vi "0x53_Write_table_data.vi"(8 "error in":errorcluster, 9 "Номер табличного параметра 2":i32, 10 "ArrayIn":sgl[][](array[numeric]), 11 "paramUnicorn":T1={"conParam"={"ReadIntParam"=TRUE, "ReadDescrParam"=FALSE, "ReadFloatParam"=TRUE, "debug"=FALSE, "ReadJSON"=TRUE, "IP_address"="192.168.1.216", "N_attempts"=3, "type_con"=enum."TCP", "MB_address"=1, "VISA"="COM1", "connection ID"=refnum, "nameDevices"="", "timeout"=3000, "port"=2000, "type_version"="0F0C0001", "baud_rate"=115200, "VersionControl"=TRUE, "TCP_conn"=TRUE, "WindowSize"=700}, "Param"={"NumParam"={"NTelem"=201, "NInt"=16, "NFloat"=10, "NTable"=2}, "ParamInt"=[{"ID"="Режим работы", "Num"=0, "Name"="", "Type"="", "Enum"="", "Desc"="", "Unit"="", "Access"="", "FormatStr"="", "Min"=0, "Max"=0}, {"ID"="", "Num"=0, "Name"="", "Type"="", "Enum"="", "Desc"="", "Unit"="", "Access"="", "FormatStr"="", "Min"=0, "Max"=0}, {"ID"="", "Num"=0, "Name"="", "Type"="", "Enum"="", "Desc"="", "Unit"="", "Access"="", "FormatStr"="", "Min"=0, "Max"=0}, {"ID"="", "Num"=0, "Name"="", "Type"="", "Enum"="", "Desc"="", "Unit"="", "Access"="", "FormatStr"="", "Min"=0, "Max"=0}, {"ID"="", "Num"=0, "Name"="", "Type"="", "Enum"="", "Desc"="", "Unit"="", "Access"="", "FormatStr"="", "Min"=0, "Max"=0}, {"ID"="", "Num"=0, "Name"="", "Type"="", "Enum"="", "Desc"="", "Unit"="", "Access"="", "FormatStr"="", "Min"=0, "Max"=0}, {"ID"="ModeWork", "Num"=0, "Name"="", "Type"="", "Enum"="", "Desc"="", "Unit"="", "Access"="", "FormatStr"="", "Min"=0, "Max"=0}], "Telemetry"=[], "Table"=[], "ParamFloat"=[]}}) -> (0 "error out":errorcluster, 2 "Ответ":string, 3 "paramUnicorn 2":T1={"conParam"={"ReadIntParam"=TRUE, "ReadDescrParam"=FALSE, "ReadFloatParam"=TRUE, "debug"=FALSE, "ReadJSON"=TRUE, "IP_address"="192.168.1.216", "N_attempts"=3, "type_con"=enum."TCP", "MB_address"=1, "VISA"="COM1", "connection ID"=refnum, "nameDevices"="", "timeout"=3000, "port"=2000, "type_version"="0F0C0001", "baud_rate"=115200, "VersionControl"=TRUE, "TCP_conn"=TRUE, "WindowSize"=700}, "Param"={"NumParam"={"NTelem"=201, "NInt"=16, "NFloat"=10, "NTable"=2}, "ParamInt"=[{"ID"="Режим работы", "Num"=0, "Name"="", "Type"="", "Enum"="", "Desc"="", "Unit"="", "Access"="", "FormatStr"="", "Min"=0, "Max"=0}, {"ID"="", "Num"=0, "Name"="", "Type"="", "Enum"="", "Desc"="", "Unit"="", "Access"="", "FormatStr"="", "Min"=0, "Max"=0}, {"ID"="", "Num"=0, "Name"="", "Type"="", "Enum"="", "Desc"="", "Unit"="", "Access"="", "FormatStr"="", "Min"=0, "Max"=0}, {"ID"="", "Num"=0, "Name"="", "Type"="", "Enum"="", "Desc"="", "Unit"="", "Access"="", "FormatStr"="", "Min"=0, "Max"=0}, {"ID"="", "Num"=0, "Name"="", "Type"="", "Enum"="", "Desc"="", "Unit"="", "Access"="", "FormatStr"="", "Min"=0, "Max"=0}, {"ID"="", "Num"=0, "Name"="", "Type"="", "Enum"="", "Desc"="", "Unit"="", "Access"="", "FormatStr"="", "Min"=0, "Max"=0}, {"ID"="ModeWork", "Num"=0, "Name"="", "Type"="", "Enum"="", "Desc"="", "Unit"="", "Access"="", "FormatStr"="", "Min"=0, "Max"=0}], "Telemetry"=[], "Table"=[], "ParamFloat"=[]}}, 5 "Сообщение об ошибке":bool)   [LabVIEW 2017, in "LV_Unicorn.lvlib"]
uses:
  LV_Unicorn.lvlib
  Control/unicorn_Param.ctl
  Control/unicorn_conn.ctl
  Control/unicorn_JSON.ctl
  Control/unicorn_ParamInt.ctl
  Control/unicorn_Telemetry.ctl
  Control/unicorn_Table.ctl
  Control/unicorn_ParamFloat.ctl
panel:
  out "Slide":u8(slide) caption="Запись табличного параметра" scale=0.0..100.0
  out "Size":i32
  out "Array":string[](array[string])
  out "length 2":i32
  out "lengthData":i32
  out "String out":string
  out "кол-во считанных байт тела запрошенного параметра":i32
  out "Начальное смещение в байтах":i32
  out "Номер табличного параметра":i32
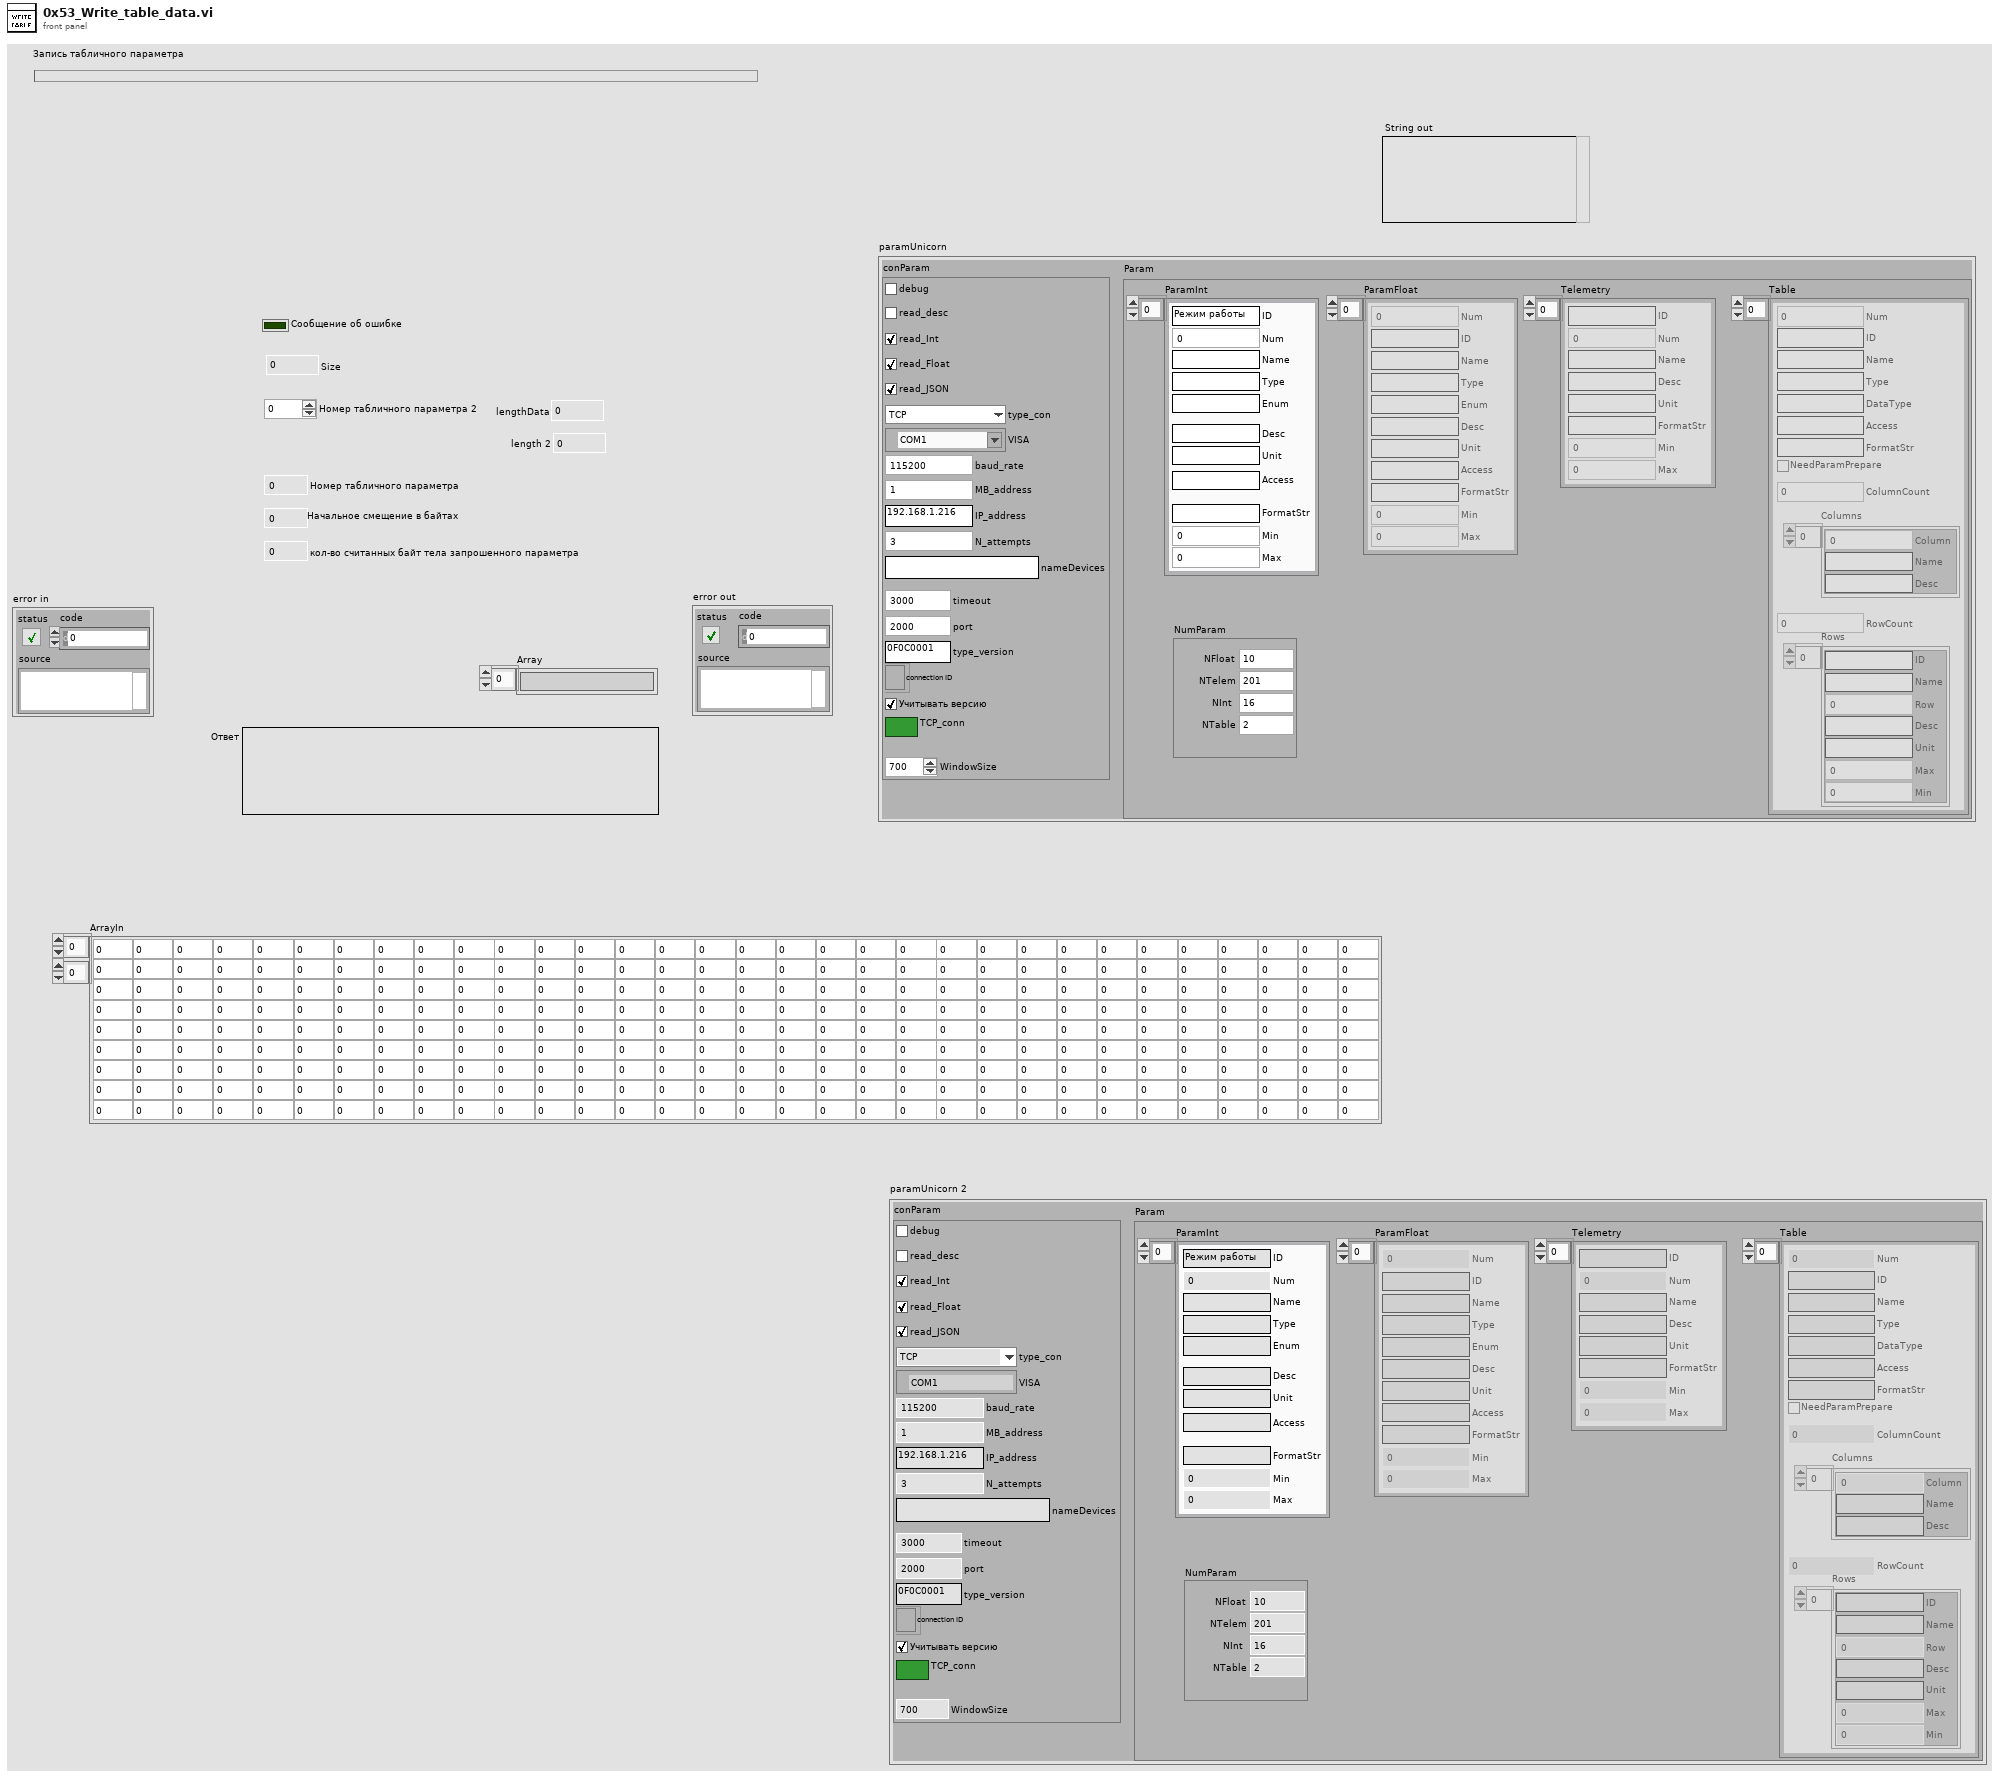
[diagram p1: front panel]
types:
  T1 = typedef "LV_Unicorn.lvlib/unicorn_Param.ctl" = cluster{"conParam":T2, "Param":T3}
  T2 = typedef "LV_Unicorn.lvlib/unicorn_conn.ctl" = cluster{"ReadIntParam":bool, "ReadDescrParam":bool, "ReadFloatParam":bool, "debug":bool, "ReadJSON":bool, "IP_address":string, "N_attempts":i32, "type_con":enum16{"Serial", "TCP"}, "MB_address":i32, "VISA":refnum<visa-resource-name>, "connection ID":refnum<k5>, "nameDevices":string, "timeout":i32, "port":u16, "type_version":string, "baud_rate":u32, "VersionControl":bool, "TCP_conn":bool, "WindowSize":i32}
  T3 = typedef "LV_Unicorn.lvlib/unicorn_JSON.ctl" = cluster{"NumParam":cluster{"NTelem":i32, "NInt":i32, "NFloat":i32, "NTable":i32}, "ParamInt":T4, "Telemetry":T5, "Table":T6, "ParamFloat":T7}
  T4 = typedef "LV_Unicorn.lvlib/unicorn_ParamInt.ctl" = cluster{"ID":string, "Num":i32, "Name":string, "Type":string, "Enum":string, "Desc":string, "Unit":string, "Access":string, "FormatStr":string, "Min":i32, "Max":i32}[]
  T5 = typedef "LV_Unicorn.lvlib/unicorn_Telemetry.ctl" = cluster{"ID":string, "Num":i32, "Name":string, "Desc":string, "Unit":string, "FormatStr":string, "Min":i32, "Max":i32}[]
  T6 = typedef "LV_Unicorn.lvlib/unicorn_Table.ctl" = cluster{"Num":i32, "Access":string, "ColumnCount":i32, "NeedParamPrepare":bool, "Columns":cluster{"Column":i32, "Desc":string, "Name":string}[], "DataType":string, "FormatStr":string, "ID":string, "Name":string, "RowCount":i32, "Rows":cluster{"Desc":string, "ID":string, "Max":i32, "Min":i32, "Name":string, "Row":i32, "Unit":string}[], "Type":string}[]
  T7 = typedef "LV_Unicorn.lvlib/unicorn_ParamFloat.ctl" = cluster{"ID":string, "Num":i32, "Name":string, "Type":string, "Enum":string, "Desc":string, "Unit":string, "Access":string, "FormatStr":string, "Min":sgl, "Max":sgl}[]
  T8 = cluster{"Начальное смещение в байтах":i32, "Номер табличного параметра":i32, "Шаг":i32, "Размер слова":i32}
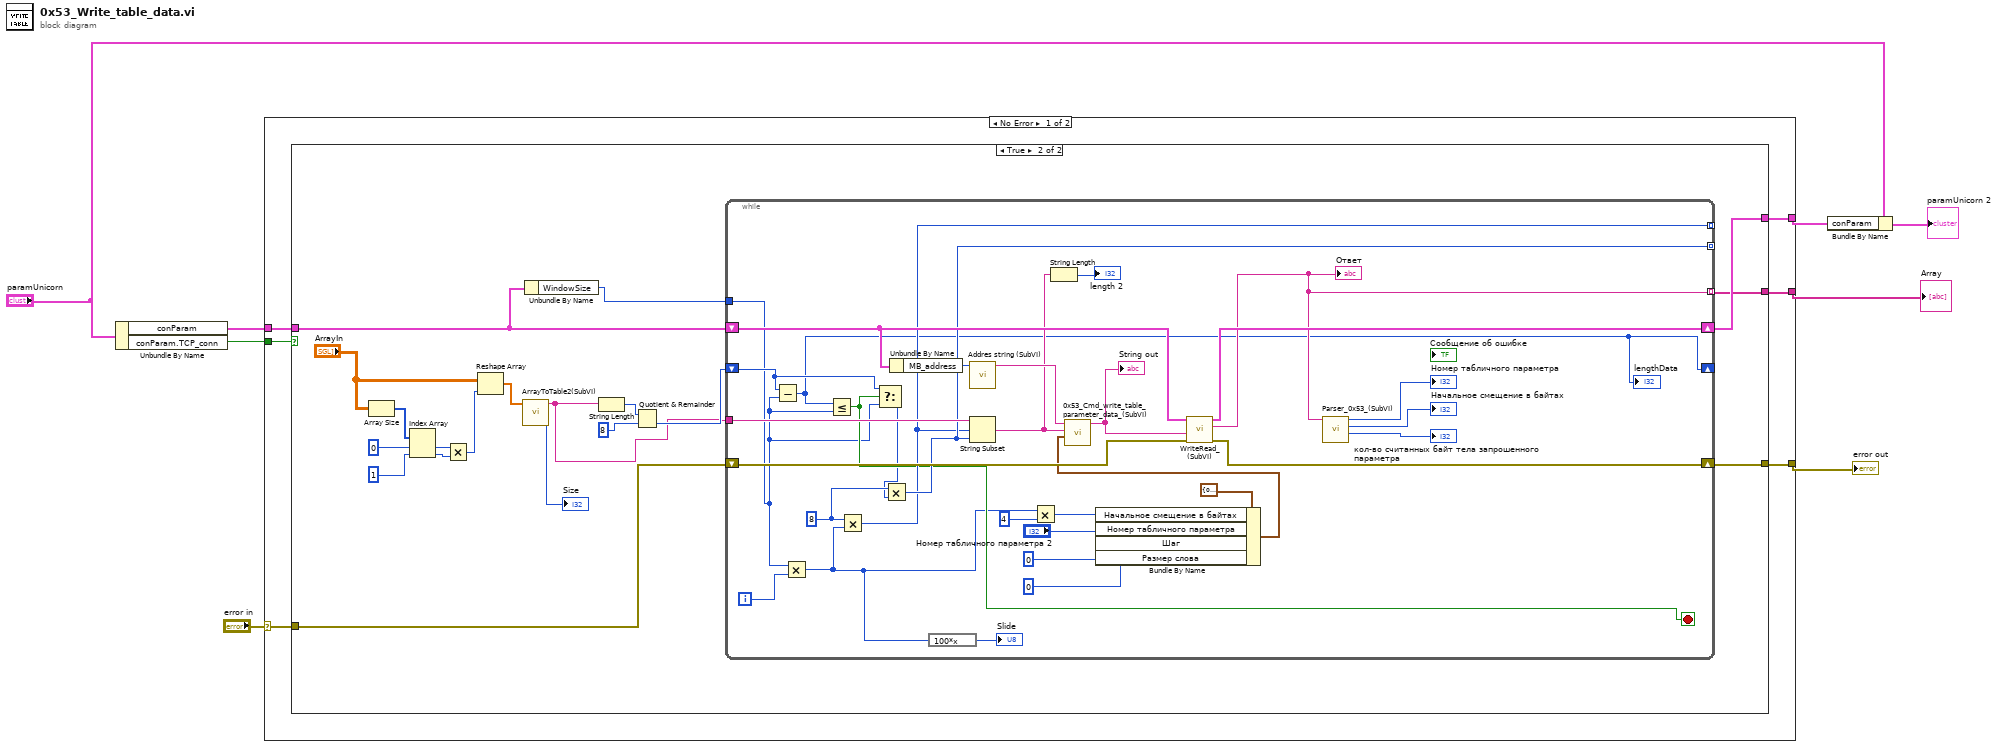
[diagram p0: block diagram]
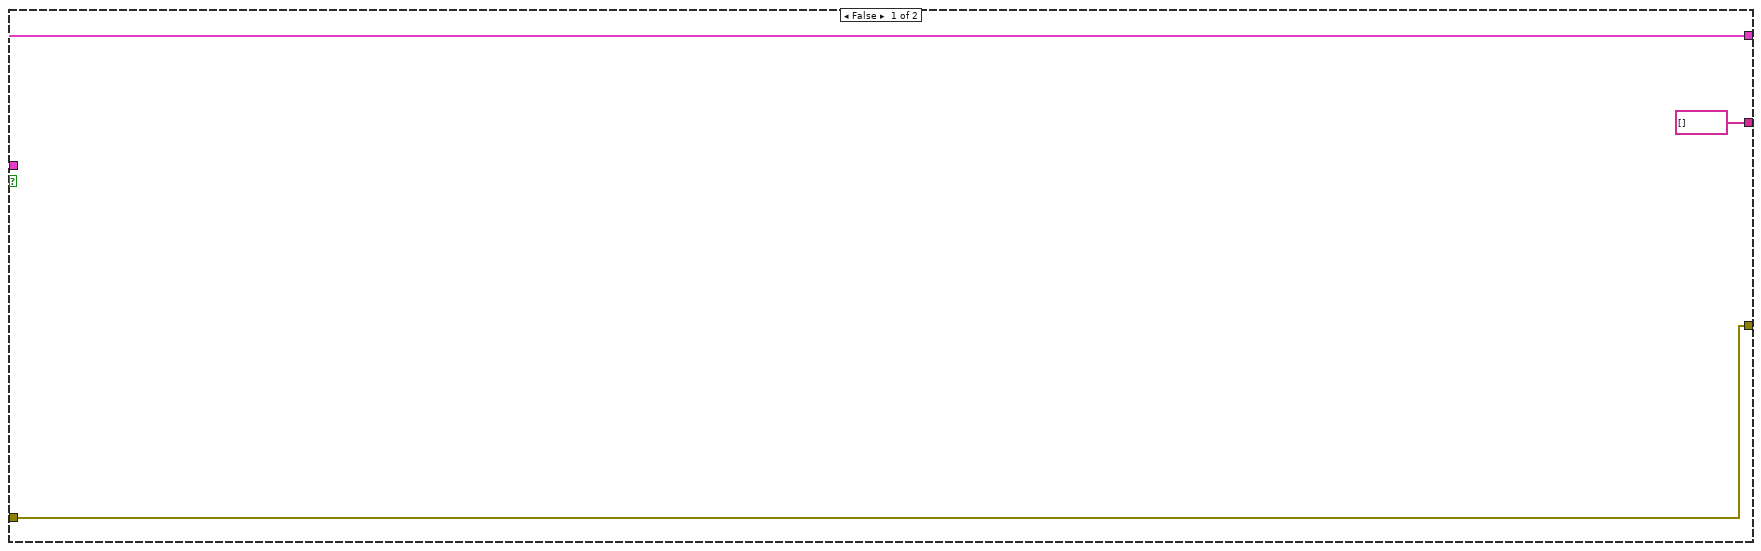
[diagram p2: hidden frame]
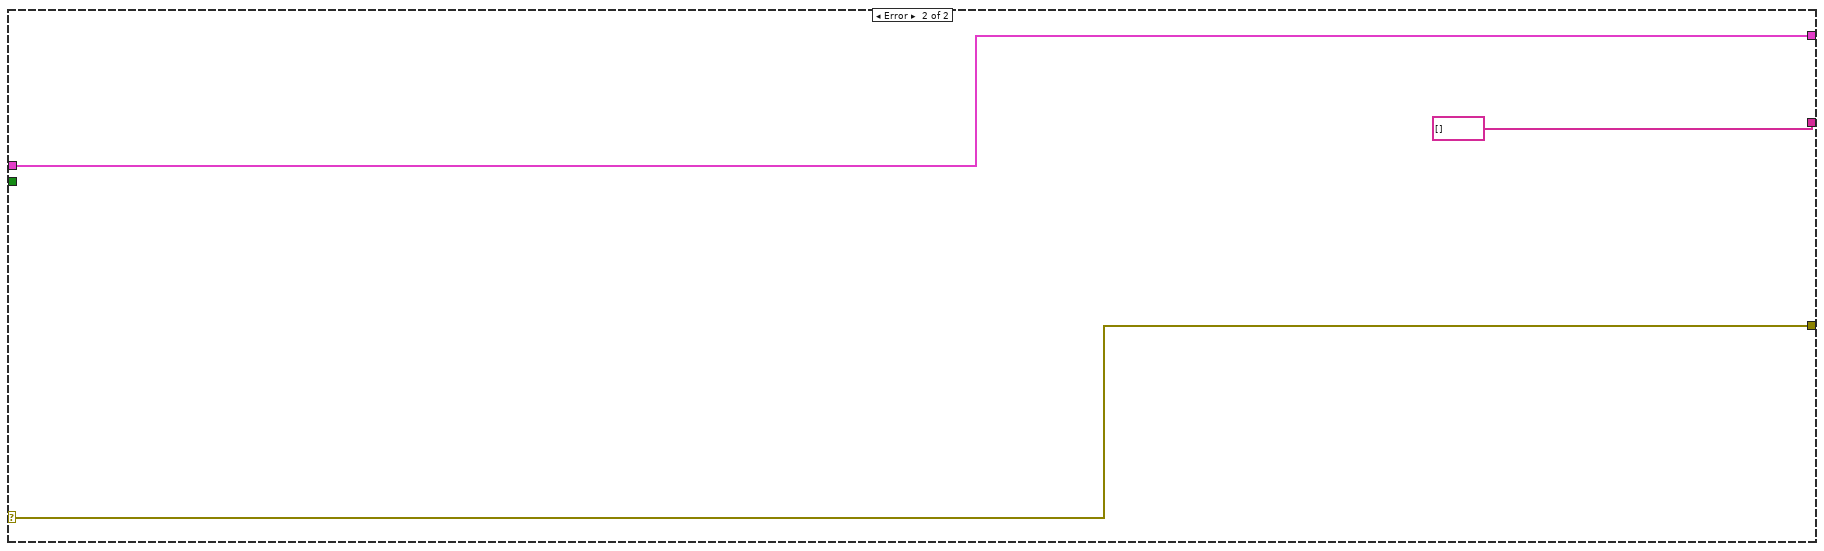
[diagram p3: hidden frame]
diagram:
  n1 = Unbundle By Name("paramUnicorn") -> ("conParam"=w6:T2, "conParam.TCP_conn"=w1:bool)
  n2 = case shown="No Error" "error in" {
    selector: "error in" -> [w12 w70]
    tunnel: w6 -> [w11 w71]
    tunnel: [w14 w71] -> w4
    tunnel: [w13 w70] -> w8
    tunnel: [w10 string[] []] -> w2
    tunnel: w1 -> [w9 _]
    frame No Error {
      n3 = case shown="True" w9 {
        tunnel: [w16 w36] -> w14
        tunnel: [w17 w35] -> w13
        tunnel: w12 -> [w17 w34]
        tunnel: w11 -> [w16 w19]
        tunnel: [string[] [] w20] -> w10
        frame False {
        }
        frame True {
          n4 = Array Size(array="ArrayIn") -> (size(s)=w30:i32[])
          n5 = Index Array(array=w30, index #1=0 ("index"), index #2=1 ("index")) -> (element #1=w31:i32, element #2=w32:i32)
          n6 = Multiply(x=w31, y=w32) -> (x*y=w33:i32)
          n7 = Reshape Array("ArrayIn", w33) -> (w28:sgl[])
          n8 = call "ArrayToTable2(SubVI).vi"("Table1D"=w28) -> ("Size"=→"Size":i32, "String"=w21:string)  [unwired: 9 in]
          n9 = Unbundle By Name(w19) -> ("WindowSize"=w18:i32)
          n10 = String Length(string=w21) -> (length=w27:i32)
          n11 = Quotient & Remainder(x=w27, y=8) -> (floor(x/y)=w22:i32)  [unwired: 1 out]
          n12 = while {
            shift-right: [w67] -> w35
            shift-left: w34 -> [w66]
            shift-right: [w68] -> w36
            shift-left: w19 -> [w65]
            tunnel: w21 -> [w59]
            tunnel: [w57] -> w20 mode=indexing
            shift-right: [w39] -> _
            shift-left: w22 -> [w43]
            tunnel: [w45] -> _ mode=indexing
            tunnel: [w50] -> _ mode=indexing
            tunnel: w18 -> [w37]
            i -> [w47]
            stop <- w44 stop-if-true
            w46 = 8 ("y")
            n13 = Subtract(x=w43, y=w37) -> (x-y=w39:i32)
            "lengthData" <- w39
            n14 = Multiply(x=w37, y=w47) -> (x*y=w38:i32)
            n15 = Less Or Equal?(x=w39, y=w37) -> (x <= y?=w44:bool)
            n16 = Multiply(x=w46, y=w38) -> (x*y=w45:i32)
            n17 = Select(t=w43, s=w44, f=w37) -> (s? t:f=w42:i32)
            n18 = Multiply(x=w46, y=w42) -> (x*y=w50:i32)
            n19 = Unbundle By Name(w65) -> ("MB_address"=w56:i32)
            n20 = expression code="100*x"(w38) -> (→"Slide":i32)
            n21 = call "Addres string (SubVI).vi"("Адрес"=w56) -> ("String"=w64:string)  [unwired: 10 in]
            n22 = String Subset(string=w59, offset (0)=w45, length (rest)=w50) -> (substring=w51:string)
            n23 = Multiply(x=w38, y=4) -> (x*y=w48:i32)
            n24 = String Length(string=w51) -> (length=→"length 2":i32)
            n25 = Bundle By Name(cluster=T8 {"Начальное смещение в байтах"=0, "Номер табличного параметра"=0, "Шаг"=0, "Размер слова"=0} ("Cluster 3"), "Начальное смещение в байтах"=w48, "Номер табличного параметра"="Номер табличного параметра 2", "Шаг"=0 ("Номер табличного параметра"), "Размер слова"=0) -> (w52:T8)
            n26 = call "0x53_Cmd_write_table_parameter_data_(SubVI).vi"("Parameters"=w52, "data"=w51, "String in"=w64) -> ("String out"=w63:string)  [unwired: 8 in]
            "String out" <- w63
            n27 = call "WriteRead_(SubVI).vi"("error in"=w66, "Запрос"=w63, "ParamIn"=w65) -> ("error out"=w67:errorcluster, "Ответ"=w57:string, "ParamOut"=w68:T2)  [unwired: 4 in, 2 out]
            "Ответ" <- w57
            n28 = call "Parser_0x53_(SubVI).vi"("String in"=w57) -> ("кол-во считанных байт тела запрошенного параметра"=→"кол-во считанных байт тела запрошенного параметра":i32, "Начальное смещение в байтах"=→"Начальное смещение в байтах":i32, "Номер табличного параметра"=→"Номер табличного параметра":i32)  [unwired: 8 in]
          }
        }
      }
    }
    frame Error {
    }
  }
  "error out" <- w8
  "Array" <- w2
  n29 = Bundle By Name(cluster="paramUnicorn", "conParam"=w4) -> (→"paramUnicorn 2":T1)
